vi "Read Data from 5772.vi"() -> ()   [LabVIEW 2011]
uses:
  <vilib>/userDefined/High Color/nirio_resource_hc.ctl
  <vilib>/FPGAPlugInAG/PXIe-7965R/niLvFpga_Open_PXIe-7965R.vi
  <vilib>/rvi/interface/common/dynamic/niFpgaDynamicAddResources.vi
  <vilib>/FPGAPlugInAG/Dynamic/niLvFpga_Run_Dynamic.vi
  <vilib>/Utility/error.llb/Error Cluster From Error Code.vi
  <vilib>/rvi/errors/niLvFpgaAdjustHostInterfaceError.vi
  <vilib>/measure/maspectr.llb/FFT Power Spectrum and PSD for 1 Chan.vi
  <vilib>/FPGAPlugInAG/Dynamic/niLvFpga_Close_Dynamic.vi
  <vilib>/rvi/interface/nirviOpenFPGA/nirviOpenFPGA.xnode
  <userlib>/Fast OCT/Debug/Version 1/FPGA Bitfiles/Current/Acquire Data from 2 channels (DRAM).lvbitx
  <vilib>/rvi/interface/nirviMethod/nirviMethod.xnode
  <vilib>/rvi/interface/nirviReadWriteControl/nirviReadWriteControl.xnode
  <vilib>/rvi/interface/nirviCloseFPGA/nirviCloseFPGA.xnode
  <userlib>/FlexRIO Host Library/FlexRIO Host Library (User).lvlib
  <vilib>/rvi/interface/Simulation/niFpgaSimulationCallBeginRW.vi
  <vilib>/measure/NI_MAPro.lvlib
  <userlib>/FlexRIO Host Library/FlexRIO Host API/Configure/Record Parameters/5772/Configure Record Parameters (5772).vi
  <vilib>/ptbypt/NI_PtbyPt.lvlib
  NiFpgaLv.dll
panel:
  out "Host FIFO Timed Out?":bool
  out "Sample Jitter":dbl format="%#_6g Samples"
  out "Phase Shift Histogram":T1(graph)
  out "detected phase (deg)":dbl format="%.2p"
  out "Detected Sine Frequency":dbl format="%.2p"
  out "FFT Size":i32
  out "FFT":cluster{"f0":dbl, "df":dbl, "magnitude":dbl[]}(graph)
  out "Channel 0 Data":i16[](graph)
  in  "Resource Name":T2
  out "NumSamplesAcquired":u32
  out "Iterations Done":i32
  in  "Stop":bool
  in  "Trigger Type":T3(ring)=enum."Software Trigger"
  in  "Record Count":u32=1
  in  "Pre Trig":u32=16
  in  "Post Trig":u32=16
  out "error out":errorcluster
  # "Gain and Offset\nFrame Trigger"
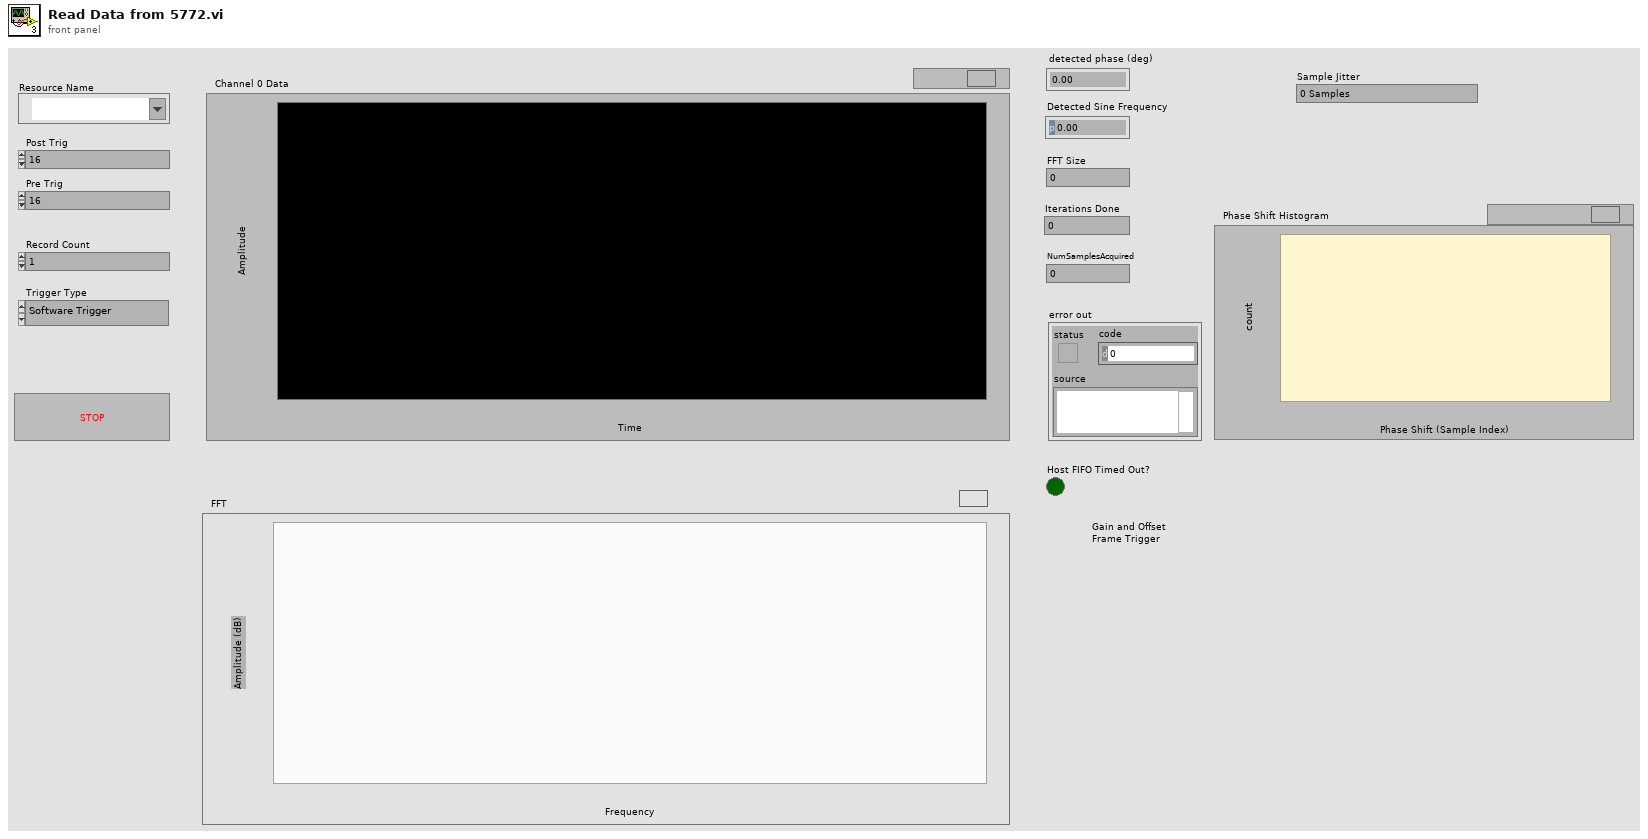
[diagram p1: front panel]
types:
  T1 = cluster{"X Values":dbl[], "Histogram: h(x)":i32[]}
  T2 = typedef "nirio_resource_hc.ctl" = tag
  T3 = enum8{"Immediate Trigger", "Software Trigger", "External Digital Trigger", "Analog Trigger"}
  T4 = cluster{"Load Record Parameters?":bool, "Pre Trigger Samples":u32, "Post Trigger Samples":u32, "Trigger Hold Off":u32, "Record Count":u32}
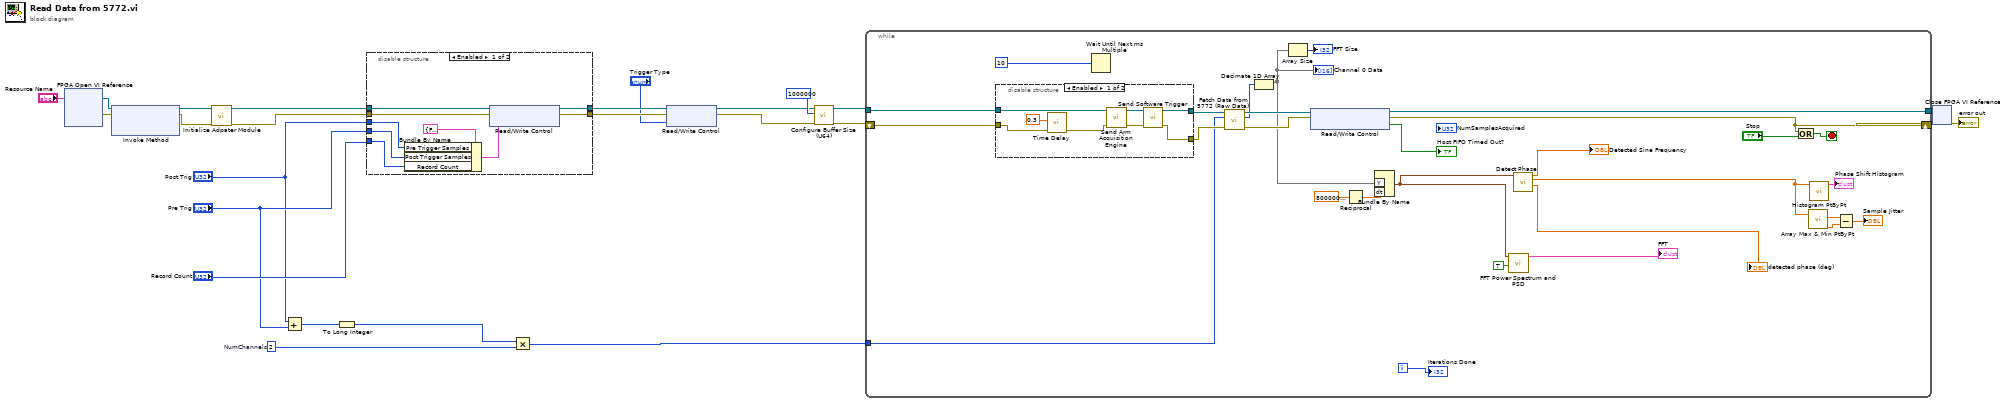
[diagram p0: block diagram]
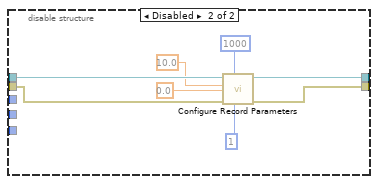
[diagram p2: hidden frame]
diagram:
  w17 = u32 2  # NumChannels
  n1 = xnode "FPGA Open VI Reference"("resource name"="Resource Name") -> ("FPGA VI Reference Out"=w15:refnum<k20>, "error out"=w12:errorcluster)  [unwired: 1 in]
  n2 = xnode "Invoke Method"("FPGA VI Reference In"=w15, "error in"=w12) -> ("FPGA VI Reference Out"=w14:refnum<k20>, "error out"=w13:errorcluster)  [unwired: 1 in]
  n3 = call <userlib>:"Initialize Adpater Module.vi"("error in"=w13, "FPGA VI Reference In"=w14) -> ("error out"=w22:errorcluster, "FPGA VI Reference Out"=w23:refnum<k20>)  [unwired: 7 in, 1 out]
  n4 = Add(x="Post Trig", y="Pre Trig") -> (x+y=w5:u32)
  n5 = To Long Integer(number=w5) -> (32bit integer=w4:i32)
  n6 = disable-structure shown="Enabled" {
    disable-tunnel: w23 -> [w34 w43]
    disable-tunnel: w22 -> [w33 w42]
    disable-tunnel: "Record Count" -> [w27 _]
    disable-tunnel: "Pre Trig" -> [w28 _]
    disable-tunnel: [w32 w40] -> w8
    disable-tunnel: [w31 w41] -> w7
    disable-tunnel: "Post Trig" -> [w29 _]
    frame Enabled {
      n7 = Bundle By Name(cluster=T4 {"Load Record Parameters?"=FALSE, "Pre Trigger Samples"=0, "Post Trigger Samples"=0, "Trigger Hold Off"=0, "Record Count"=0} ("Record Parameters"), "Pre Trigger Samples"=w29, "Post Trigger Samples"=w28, "Record Count"=w27) -> (w26:T4)
      n8 = xnode "Read/Write Control"("FPGA VI Reference In"=w34, "error in"=w33, "Record Parameters"=w26) -> ("FPGA VI Reference Out"=w32:refnum<k20>, "error out"=w31:errorcluster)
    }
    frame Disabled {
      n9 = call-poly <userlib>:"Configure Record Parameters.vi"("Record Count"=u16 1, "Record Length"=u16 1000, "error in"=w42, "% of Acquisition Hold Off Time"=0.0, "% of Pre-Trigger Samples"=10.0, "FPGA VI Reference In"=w43) -> ("error out"=w41:errorcluster, "FPGA VI Reference Out"=w40:refnum<k20>, "Actual Record Length"=w37:u16)  [unwired: 3 in]
    }
  }
  n10 = Multiply(x=w4, y=w17) -> (x*y=w16:u32)
  n11 = xnode "Read/Write Control"("FPGA VI Reference In"=w8, "error in"=w7, "Trigger Type"="Trigger Type") -> ("FPGA VI Reference Out"=w1:refnum<k20>, "error out"=w2:errorcluster)
  n12 = call <userlib>:"Configure Buffer Size (U64).vi"("error in"=w2, "Buffer Size"=u32 1000000, "FPGA VI Reference In"=w1) -> ("error out"=w10:errorcluster, "FPGA VI Reference Out"=w11:refnum<k20>)  [unwired: 7 in]
  n13 = while {
    shift-right: [w68] -> w19
    shift-left: w10 -> [w44]
    tunnel: w11 -> [w45]
    tunnel: [w69] -> w20
    tunnel: w16 -> [w57]
    i -> [w67]
    stop <- w71 stop-if-true
    n14 = disable-structure shown="Enabled" {
      disable-tunnel: w45 -> [w80 w82]
      disable-tunnel: w44 -> [w74 w81]
      disable-tunnel: [w76 w82] -> w46
      disable-tunnel: [w77 w81] -> w66
      frame Enabled {
        n15 = call "Time Delay"("error in (no error)"=w74, "Delay Time (s)"=0.3) -> ("error out"=w73:errorcluster)  [unwired: 9 in]
        n16 = call <userlib>:"Send Arm Acquisition Engine.vi"("error in"=w73, "FPGA VI Reference In"=w80) -> ("error out"=w78:errorcluster, "FPGA VI Reference Out"=w79:refnum<k20>)  [unwired: 8 in]
        n17 = call <userlib>:"Send Software Trigger.vi"("error in"=w78, "FPGA VI Reference In"=w79) -> ("error out"=w77:errorcluster, "FPGA VI Reference Out"=w76:refnum<k20>)  [unwired: 8 in]
      }
      frame Disabled {
      }
    }
    n18 = Wait Until Next ms Multiple(millisecond multiple=u32 10) -> ()  [unwired: 1 out]
    n19 = call <userlib>:"Fetch Data from 5772 (Raw Data).vi"("error in"=w66, "Samples"=w57, "FPGA VI Reference In"=w46) -> ("error out"=w64:errorcluster, "Data Acquired"=w50:i16[], "FPGA VI Reference Out"=w65:refnum<k20>)  [unwired: 6 in]
    n20 = Decimate 1D Array(w50) -> (w48:i16[])  [unwired: 1 out]
    "Channel 0 Data" <- w48
    n21 = Array Size(array=w48) -> (size(s)=→"FFT Size":i32)
    n22 = xnode "Read/Write Control"("FPGA VI Reference In"=w65, "error in"=w64) -> ("FPGA VI Reference Out"=w69:refnum<k20>, "error out"=w68:errorcluster, "Host FIFO Timed Out?"=→"Host FIFO Timed Out?":bool)
    n23 = Reciprocal(x=800000000.0) -> (1/x=w62:dbl)
    n24 = Bundle By Name("Y"=w48, "dt"=w62) -> (w58:waveform(i16))  [unwired: 1 in]
    n25 = call-poly <vilib>:"FFT Power Spectrum and PSD.vi"("dB On (F)"=TRUE, "time signal"=w58) -> ("Power Spectrum / PSD"=→"FFT":cluster{"f0":dbl, "df":dbl, "magnitude":dbl[]})  [unwired: 6 in, 3 out]
    n26 = call <userlib>:"Detect Phase.vi"("Input Wavceform"=w58) -> ("Phase in Degress"=→"detected phase (deg)":dbl, "Phase in Samples"=w51:dbl, "Detected Sine Frequency"=→"Detected Sine Frequency":dbl)  [unwired: 8 in]
    n27 = Compound Arithmetic op=OR(w68, "Stop") -> (w71:bool)
    n28 = call <vilib>:"Array Max & Min PtByPt.vi"("input data point"=w51) -> ("max value"=w55:dbl, "min value"=w54:dbl)  [unwired: 2 in, 3 out]
    n29 = call <vilib>:"Histogram PtByPt.vi"("x"=w51) -> ("Histogram Graph"=→"Phase Shift Histogram":T1)  [unwired: 7 in, 3 out]
    n30 = Subtract(x=w55, y=w54) -> (x-y=→"Sample Jitter":dbl)
    "Iterations Done" <- w67
  }
  n31 = xnode "Close FPGA VI Reference"("FPGA VI Reference In"=w20, "error in"=w19) -> ("error out"=→"error out":errorcluster)
